vi "DataProcessing.vi"(0 "queue in":refnum<queue>, 1 "element":u8, 2 "error in":errorcluster) -> (3 "queue out":refnum<queue>, 4 "Boolean":bool=TRUE, 5 "Message out":T1={"Timestamp(4)"=0, "Sequence(4)"=0, "JY61ACC(2)"=[], "JY61GRY(3)"=[], "JY61AGL(3)"=[], "GY52ACC(2)"=[], "GY52GRY(3)"=[], "ADC1(3)"=[], "ADC2(3)"=[], "LFT/RAT"="DIR"}, 6 "error out":errorcluster)   [LabVIEW 2014]
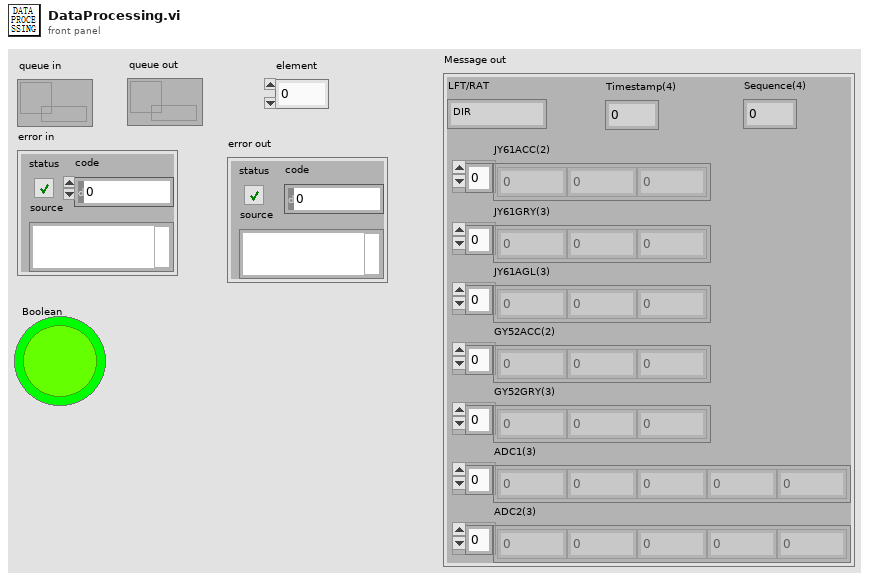
[diagram p1: front panel]
types:
  T1 = cluster{"Timestamp(4)":u32, "Sequence(4)":u32, "JY61ACC(2)":dbl[], "JY61GRY(3)":dbl[], "JY61AGL(3)":dbl[], "GY52ACC(2)":dbl[], "GY52GRY(3)":dbl[], "ADC1(3)":dbl[], "ADC2(3)":dbl[], "LFT/RAT":string}
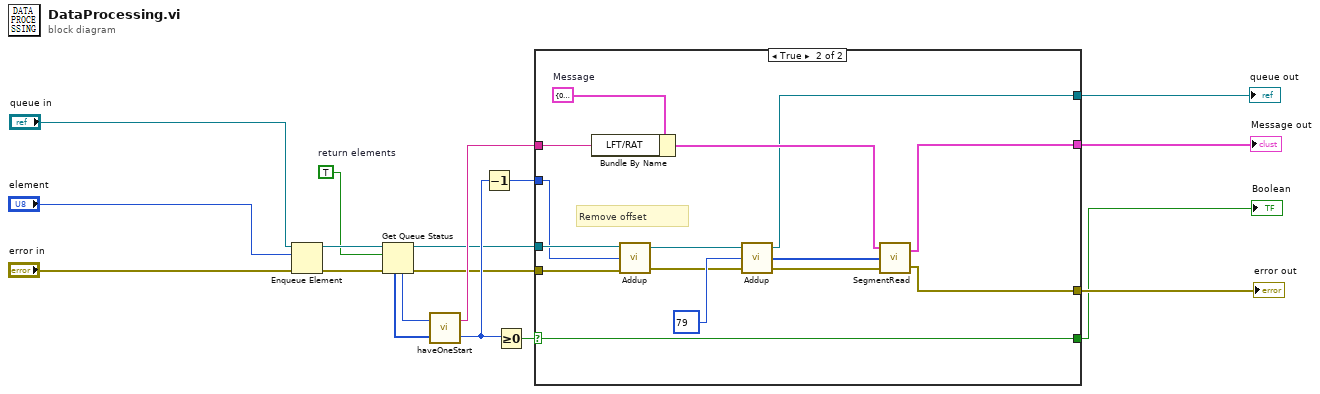
[diagram p0: block diagram]
diagram:
  w15 = TRUE  # return elements
  n1 = Enqueue Element(queue="queue in", element="element", error in (no error)="error in") -> (queue out=w16:refnum<queue>, error out=w17:errorcluster)  [unwired: 1 in, 1 out]
  n2 = Get Queue Status(queue=w16, return elements? (F)=w15, error in (no error)=w17) -> (queue out=w9:refnum<queue>, error out=w8:errorcluster, # elements in queue=w13:i32, elements=w14:u8[])  [unwired: 4 out]
  n3 = call "haveOneStart.vi"("Byte Array"=w14, "Length"=w13) -> ("offset"=w11:i32, "match substring"=w10:string)
  n4 = Decrement(x=w11) -> (x-1=w18:i32)
  n5 = Greater Or Equal To 0?(x=w11) -> (x >= 0?=w12:bool)
  n6 = case shown="True" w12 {
    selector: w12 -> [w21 w25]
    tunnel: w18 -> [_ w32]
    tunnel: w10 -> [_ w35]
    tunnel: w9 -> [w19 w34]
    tunnel: w8 -> [w20 w33]
    tunnel: [w21 w25] -> w2
    tunnel: [_ w24] -> w5
    tunnel: [w20 w23] -> w3
    tunnel: [w19 w22] -> w6
    frame False {
    }
    frame True {
      w36 = T1 {"Timestamp(4)"=0, "Sequence(4)"=0, "JY61ACC(2)"=[], "JY61GRY(3)"=[], "JY61AGL(3)"=[], "GY52ACC(2)"=[], "GY52GRY(3)"=[], "ADC1(3)"=[], "ADC2(3)"=[], "LFT/RAT"="DIR"}  # Message
      # "Remove offset"
      n7 = Bundle By Name(cluster=w36, "LFT/RAT"=w35) -> (w26:T1)
      n8 = call "Addup.vi"("error in (no error)"=w33, "Length"=w32, "queue in"=w34) -> ("error out"=w29:errorcluster, "queue out"=w30:refnum<queue>)  [unwired: 1 out]
      n9 = call "Addup.vi"("error in (no error)"=w29, "Length"=79, "queue in"=w30) -> ("error out"=w28:errorcluster, "Byte Array"=w27:u8[], "queue out"=w22:refnum<queue>)
      n10 = call "SegmentRead.vi"("error in"=w28, "Byte Array"=w27, "Input Message"=w26) -> ("error out"=w23:errorcluster, "Output Message"=w24:T1)
    }
  }
  "error out" <- w3
  "Message out" <- w5
  "queue out" <- w6
  "Boolean" <- w2
